vi "MAX31855USB_get_val.vi"(4 "error in (no error)":errorcluster, 7 "VISA resource name":refnum<visa-resource-name>) -> (0 "error out":errorcluster, 1 "array":dbl[](array[numeric]), 3 "VISA resource name out":refnum<visa-resource-name>)   [LabVIEW 2014]
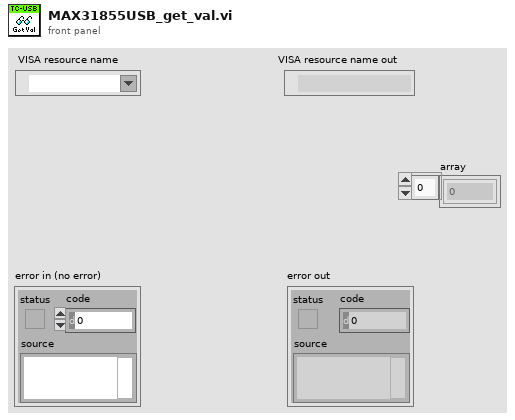
[diagram p1: front panel]
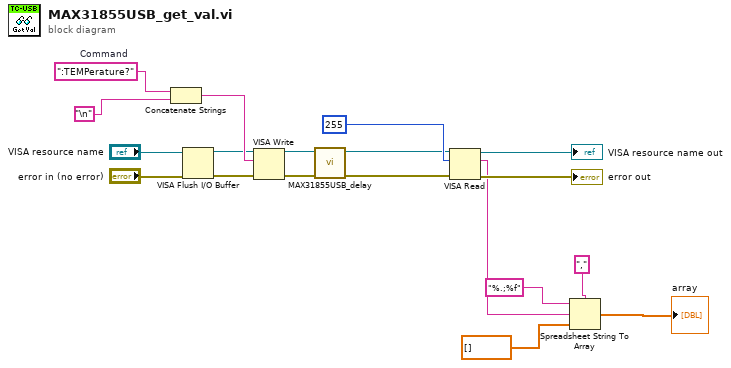
[diagram p0: block diagram]
diagram:
  w12 = ":TEMPerature?"  # Command
  n1 = Concatenate Strings(w12, "\n") -> (w17:string)
  n2 = VISA Flush I/O Buffer(VISA resource name="VISA resource name", error in (no error)="error in (no error)") -> (VISA resource name out=w15:refnum<visa-resource-name>, error out=w16:errorcluster)  [unwired: 1 in]
  n3 = VISA Write(VISA resource name=w15, write buffer=w17, error in (no error)=w16) -> (VISA resource name out=w19:refnum<visa-resource-name>, error out=w18:errorcluster)  [unwired: 1 out]
  n4 = call "MAX31855USB_delay.vi"("error in (no error)"=w18, "VISA Refnum in"=w19) -> ("error out"=w6:errorcluster, "VISA Refnum out"=w7:refnum<visa-resource-name>)  [unwired: 8 in]
  n5 = VISA Read(VISA resource name=w7, byte count=u32 255 ("Byte-Anzahl"), error in (no error)=w6) -> (VISA resource name out=→"VISA resource name out":refnum<visa-resource-name>, read buffer=w4:string, error out=→"error out":errorcluster)  [unwired: 1 out]
  n6 = Spreadsheet String To Array(delimiter (Tab)=",", format string="%.;%f", spreadsheet string=w4, array type (2D Dbl)=dbl[] []) -> (array=→"array":dbl[])
